vi "G# - Polymorphism demo2.vi"() -> ()   [LabVIEW 2020]
doc: "Polymorphism - Error in casting\nThis demo will show polymorphism in action. Three objects are created and the references are casted to DemoSubClass1 type.\nThe last casting will fail since DemoClass1 could not be casted to the more specific DemoSubClass1.\n\nBy using the G# Debugger found in Tools->G# Debugger a text log can be followed showing how the objects were created and destroyed."
uses:
  DemoSubClass1_class/DemoSubClass1.lvclass
  DemoSubSubClass1_class/DemoSubSubClass1.lvclass
  DemoClass1_class/DemoClass1.lvclass
  <vilib>/addons/_AddQ/G#Object/G#Object.lvclass
panel:
  in  "error in (no error)":errorcluster
  out "error out":errorcluster
  # "Polymorphism - Error in casting\nThis demo will show polymorphism in action. Three objects are created and the references are casted to DemoSubClass1 type.\nThe last casting will fail since DemoClass1 could not be casted to the more specific DemoSubClass1.\n\nBy using the G# Debugger found in Tools->G# Debugger a text log can be followed showing how the objects were created and destroyed."
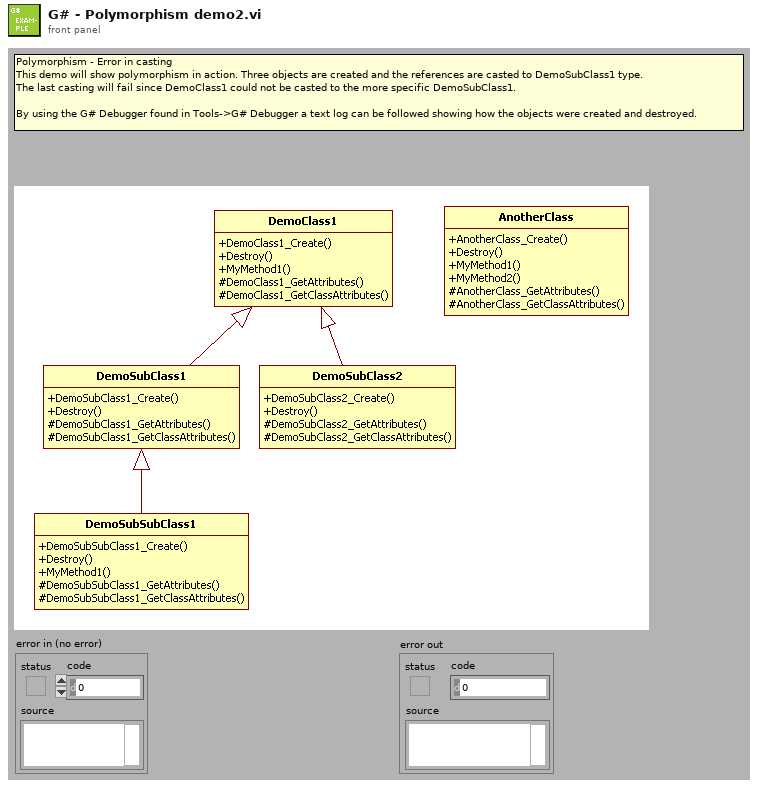
[diagram p1: front panel]
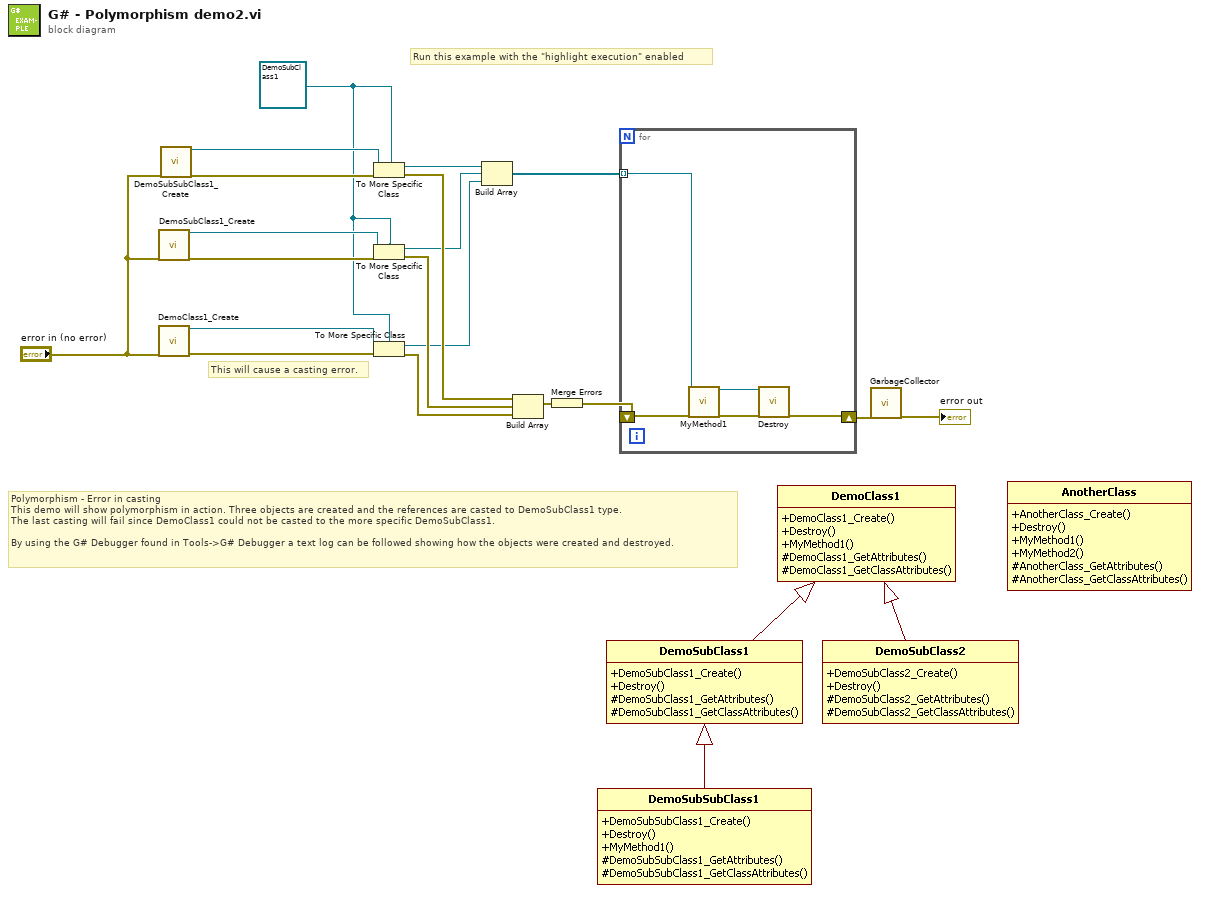
[diagram p0: block diagram]
diagram:
  w8 = refnum<class "DemoSubClass1.lvclass"> refnum ("reference out")
  # "Polymorphism - Error in casting\nThis demo will show polymorphism in action. Three objects are created and the references are casted to DemoSubClass1 type.\nThe last casting will fail since DemoClass1 could not be casted to the more specific DemoSubClass1.\n\nBy using the G# Debugger found in Tools->G# Debugger a text log can be followed showing how the objects were created and destroyed."
  # "Run this example with the \"highlight execution\" enabled"
  # "This will cause a casting error."
  n1 = call "DemoSubClass1_Create.vi"("error in (no error)"="error in (no error)") -> ("reference out"=w14:refnum<class "DemoSubClass1.lvclass">, "error out"=w15:errorcluster)  [unwired: 17 out]
  n2 = call "DemoClass1_Create.vi"("error in (no error)"="error in (no error)") -> ("reference out"=w9:refnum<class "DemoClass1.lvclass">, "error out"=w10:errorcluster)  [unwired: 17 out]
  n3 = call "DemoSubSubClass1_Create.vi"("error in (no error)"="error in (no error)") -> ("reference out"=w16:refnum<class "DemoSubSubClass1.lvclass">, "error out"=w17:errorcluster)  [unwired: 17 out]
  n4 = To More Specific Class(target class=w8, reference=w16, error in=w17) -> (specific class reference=w7:refnum<class "DemoSubClass1.lvclass">, error out=w13:errorcluster)
  n5 = To More Specific Class(target class=w8, reference=w14, error in=w15) -> (specific class reference=w6:refnum<class "DemoSubClass1.lvclass">, error out=w12:errorcluster)
  n6 = To More Specific Class(target class=w8, reference=w9, error in=w10) -> (specific class reference=w5:refnum<class "DemoSubClass1.lvclass">, error out=w11:errorcluster)
  n7 = Build Array(w7, w6, w5) -> (w4:refnum<class "DemoSubClass1.lvclass">[])
  n8 = Build Array(w13, w12, w11) -> (w19:errorcluster[])
  n9 = Merge Errors(w19) -> (w18:errorcluster)
  n10 = for {
    tunnel: w4 -> [w23] mode=indexing
    shift-right: [w21] -> w3
    shift-left: w18 -> [w24]
    n11 = call-dynamic "MyMethod1.vi"("reference in"=w23, "error in (no error)"=w24) -> ("reference out"=w20:refnum<class "DemoSubClass1.lvclass">, "error out"=w22:errorcluster)  [unwired: 16 out]
    n12 = call-dynamic "Destroy.vi"("reference in"=w20, "error in (no error)"=w22) -> ("error out"=w21:errorcluster)  [unwired: 17 out]
  }
  n13 = call <vilib>:"GarbageCollector.vi"("error in (no error)"=w3) -> ("error out"=→"error out":errorcluster)  [unwired: 16 in, 2 out]
